vi "Terminal-PressureSystem-LubricateUnit-SwitchSetter.vi"(8 "error in (no error)":errorcluster caption="错误输入（无错误）", 10 "启停":bool=TRUE, 11 "operation timeout (ms)":i32=5000 caption="操作超时（5000毫秒）") -> (0 "error out":errorcluster caption="错误输出")   [LabVIEW 2014]
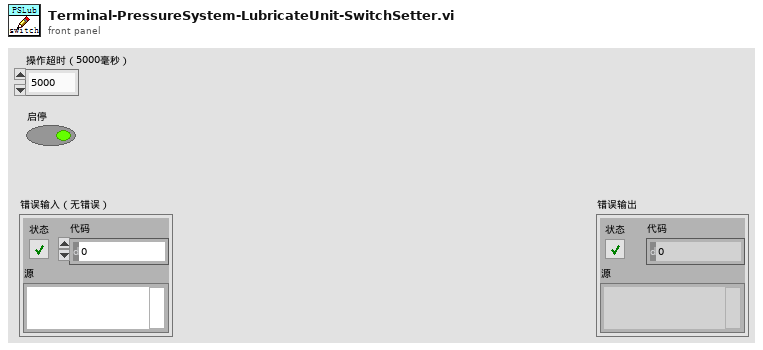
[diagram p1: front panel]
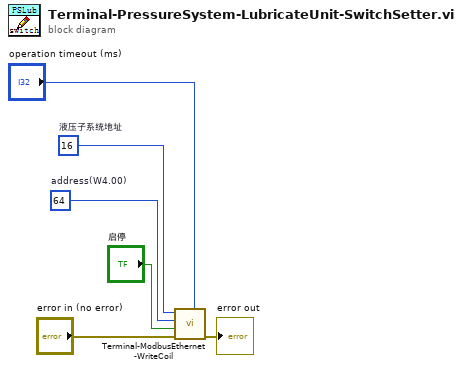
[diagram p0: block diagram]
diagram:
  w3 = u16 64  # address(W4.00)
  w4 = u8 16  # 液压子系统地址
  n1 = call "Terminal-ModbusEthernet-WriteCoil.vi"("write operation timeout (ms)"="operation timeout (ms)", "error in"="error in (no error)", "coil value"="启停", "address"=w3, "unit ID"=w4) -> ("error out"=→"error out":errorcluster)  [unwired: 6 in]
